vi "Navigate - Base VI For Navigation.vi"(1 "Curr Mining Run":i32=3, 2 "Pathfinding Settings":T1={"Movement Settings"={"Arrival Tolerance (m)"=0.05, "Closeness Threshold (m)"=0.5, "Pit Obstacle Radius (m)"=0.4, "Pit Locations"=[]}, "Dead Zone"=0.9, "Max Moves"=4.0, "Move Segment Length (m)"=0.2, "Path Cost Weights"={"Length Weight"=1.0, "Angle Weight"=0.0, "Angle Error Weight"=150.0, "Angle Error Threshold"=1.04, "Per Move Penalty"=0.25, "Closeness Weight"=3.0, "Too Short Penalty"=100.0, "Too Short Threshold"=1.75}, "Desperation - Reduction Per Attempt (Ratio)"=0.9, "Desperation - Max Attempts"=2, "Log All Move Points"=FALSE, "Intermediate Position Grids"=[{"x1"=0.0, "x2"=4.75, "resolution"=0.45}]}, 3 "Move Type":T5(ring)=enum."Move To Collector Trough") -> ()   [LabVIEW 2015, in "Navigation2017.lvlib"]
uses:
  Navigation2017.lvlib
  PathfindingSettings.ctl
  MovementSettings.ctl
  PathCostWeights.ctl
  IntermediatePositionGrids.ctl
  Vector.ctl
  LocalizationStatus.ctl
  <vilib>/Analysis/coordinate.llb/Angle Units.ctl
  PathOfMoves.ctl
  Move.ctl
  <vilib>/Analysis/coordinate.llb/Absolute Angle Difference (scalar).vi
  <vilib>/Analysis/coordinate.llb/Wrap Angle (scalar).vi
  <vilib>/Analysis/coordinate.llb/Set Angle Unit.vi
  Types - Navigation2017.lvlib
  SubVIs - Navigation2017.lvlib
  Util - Navigation2017.lvlib
  TestbenchUtils - Navigation2017.lvlib
  <vilib>/Analysis/NI_AAL_Angle.lvlib
panel:
  in  "Reached Next Path Point Threshold Angle (rad)":dbl(knob)=1.5491432484410714 scale=0.0..3.14
  out "Pathfinding Loop Count":i32=1
  in  "Reached Next Path Point Threshold Distance (m)":dbl(knob)=0.4892209620058784 scale=0.0..1.0
  in  "Robot Speed":dbl(slide)=1.0 scale=0.0..1.0
  in  "Dead Reckoning Move Distance (m)":dbl(knob)=1.4397205209376083 scale=0.5..4.0
  in  "Turning Radius (m)":dbl(knob)=2.2057844750732873 scale=0.75..4.0
  # "NOTE: Log All Move Points is ignored and\nautomatically switched off."
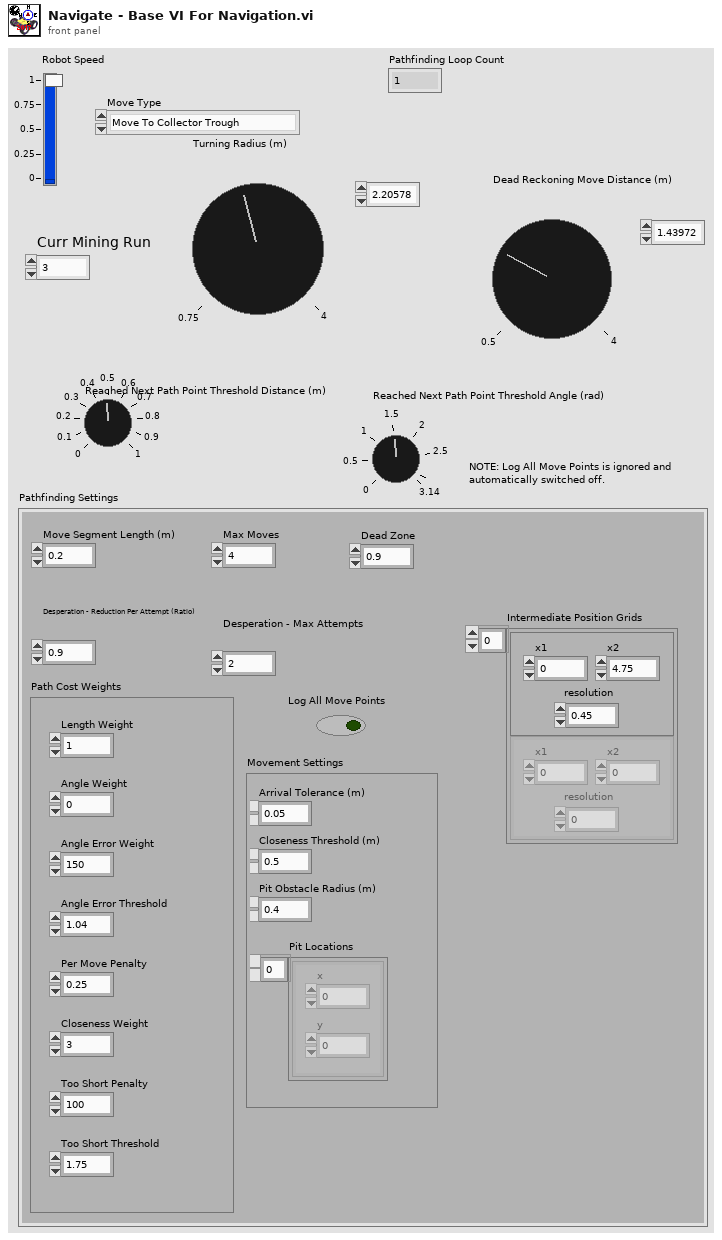
[diagram p1: front panel]
types:
  T1 = typedef "Navigation2017.lvlib/Types - Navigation2017.lvlib/PathfindingSettings.ctl" = cluster{"Movement Settings":T2, "Dead Zone":dbl, "Max Moves":dbl, "Move Segment Length (m)":dbl, "Path Cost Weights":T3, "Desperation - Reduction Per Attempt (Ratio)":dbl, "Desperation - Max Attempts":i16, "Log All Move Points":bool, "Intermediate Position Grids":T4}
  T2 = typedef "Navigation2017.lvlib/Types - Navigation2017.lvlib/MovementSettings.ctl" = cluster{"Arrival Tolerance (m)":dbl, "Closeness Threshold (m)":dbl, "Pit Obstacle Radius (m)":dbl, "Pit Locations":cluster{"x":dbl, "y":dbl}[]}
  T3 = typedef "Navigation2017.lvlib/Types - Navigation2017.lvlib/PathCostWeights.ctl" = cluster{"Length Weight":dbl, "Angle Weight":dbl, "Angle Error Weight":dbl, "Angle Error Threshold":dbl, "Per Move Penalty":dbl, "Closeness Weight":dbl, "Too Short Penalty":dbl, "Too Short Threshold":dbl}
  T4 = typedef "Navigation2017.lvlib/Types - Navigation2017.lvlib/IntermediatePositionGrids.ctl" = cluster{"x1":dbl, "x2":dbl, "resolution":dbl}[]
  T5 = enum16{"Spin and Move To Mining Area", "Move To Collector Trough", "Move To Mining Area"}
  T6 = typedef "Navigation2017.lvlib/Types - Navigation2017.lvlib/Vector.ctl" = cluster{"x":dbl, "y":dbl, "angle":dbl}
  T7 = typedef "Navigation2017.lvlib/TestbenchUtils - Navigation2017.lvlib/LocalizationStatus.ctl" = cluster{"x":dbl, "y":dbl, "angle":dbl, "valid":bool, "lastUpdatedTime":dbl}
  T8 = typedef "Navigation2017.lvlib/Types - Navigation2017.lvlib/PathOfMoves.ctl" = cluster{"Dest Angle Error":dbl, "Dest Angle Considered":bool, "Moves":T9[]}
  T9 = typedef "Navigation2017.lvlib/Types - Navigation2017.lvlib/Move.ctl" = cluster{"Did Reach Dest":bool, "Did Collide":bool, "Sum of Angle Changes (rad)":dbl, "Move Length (m)":dbl, "Closeness Sum":dbl, "Positions Along Move":T6[], "Moved Fwd":bool}
  T10 = typedef "NI_AAL_Angle.lvlib/Angle Units.ctl" = i32
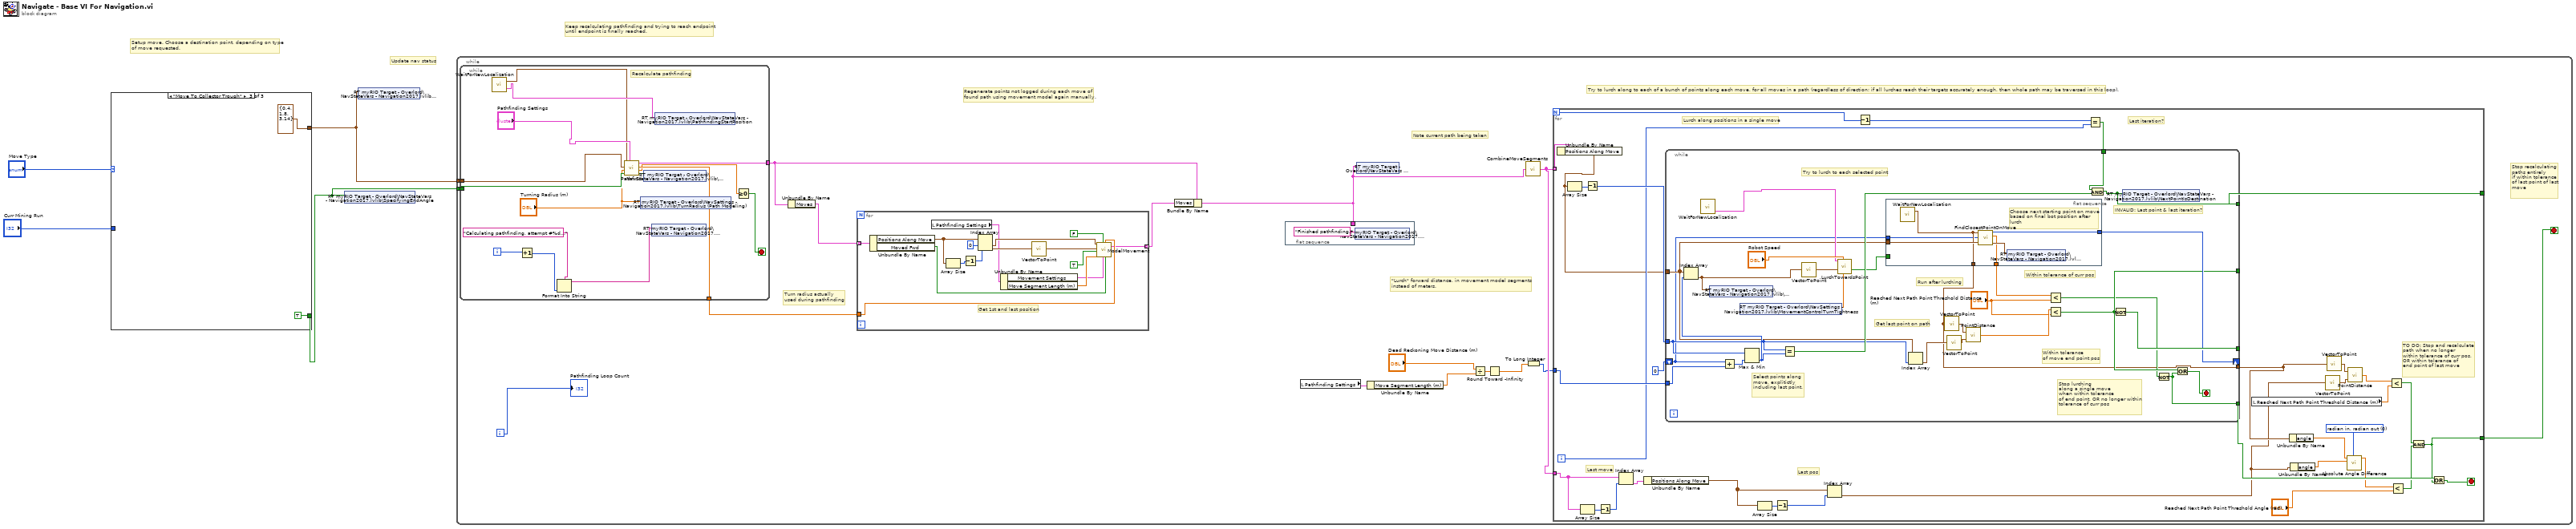
[diagram p0: block diagram]
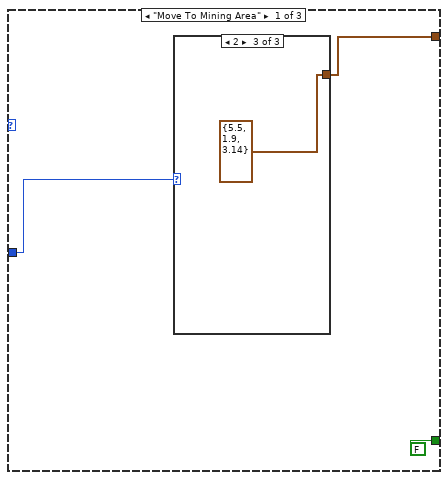
[diagram p2: hidden frame]
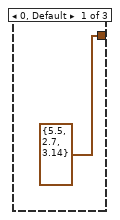
[diagram p3: hidden frame]
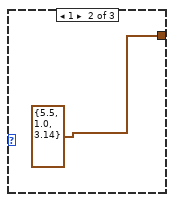
[diagram p4: hidden frame]
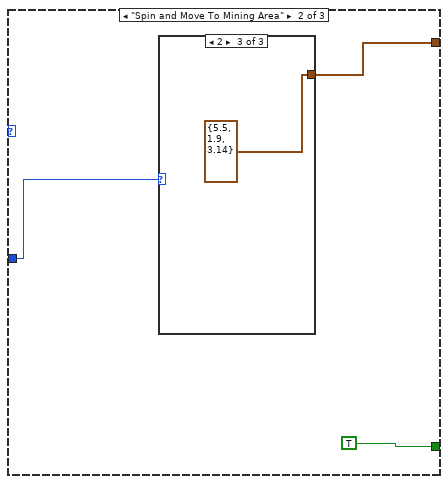
[diagram p5: hidden frame]
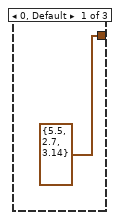
[diagram p6: hidden frame]
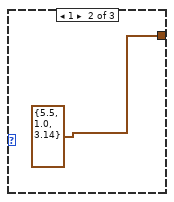
[diagram p7: hidden frame]
diagram:
  # "Keep recalculating pathfinding and trying to reach endpoint\nuntil endpoint is finally reached."
  # "Update nav status"
  # "Setup move. Choose a destination point, depending on type\nof move requested."
  n1 = case shown="\"Move To Collector Trough\"" "Move Type" {
    tunnel: [w5 w12 T6 {"x"=0.4, "y"=1.8, "angle"=3.14} ("Vector")] -> w3
    tunnel: [FALSE TRUE TRUE] -> w2
    tunnel: "Curr Mining Run" -> [w6 w11 _]
    frame "Move To Mining Area" {
      n2 = case shown="2" w6 {
        tunnel: [T6 {"x"=5.5, "y"=2.7, "angle"=3.14} ("Vector") T6 {"x"=5.5, "y"=1.0, "angle"=3.14} ("Vector") T6 {"x"=5.5, "y"=1.9, "angle"=3.14} ("Vector")] -> w5
        frame 0, Default {
        }
        frame 1 {
        }
        frame 2 {
        }
      }
    }
    frame "Spin and Move To Mining Area" {
      n3 = case shown="2" w11 {
        tunnel: [T6 {"x"=5.5, "y"=2.7, "angle"=3.14} ("Vector") T6 {"x"=5.5, "y"=1.0, "angle"=3.14} ("Vector") T6 {"x"=5.5, "y"=1.9, "angle"=3.14} ("Vector")] -> w12
        frame 0, Default {
        }
        frame 1 {
        }
        frame 2 {
        }
      }
    }
    frame "Move To Collector Trough" {
    }
  }
  n4 = shared-variable "RT myRIO Target - Overlord\\NavStateVars - Navigation2017.lvlib\\SpecifyingEndAngle"(w2) -> ()  [unwired: 1 in, 1 out]
  n5 = shared-variable "RT myRIO Target - Overlord\\NavStateVars - Navigation2017.lvlib\\DestinationPoint"(w3) -> ()  [unwired: 1 in, 1 out]
  n6 = while {
    tunnel: w3 -> [w33]
    tunnel: w2 -> [w32]
    i -> [w34]
    stop <- w21 stop-if-true
    # "Stop recalculating\npaths entirely\nif within tolerance\nof last point of last\nmove"
    # "Try to lurch along to each of a bunch of points along each move, for all moves in a path (regardless of direction; if all lurches reach their targets accurately enough, then whole path may be traversed in this loop)."
    # "Turn radius actually\nused during pathfinding"
    # "Regenerate points not logged during each move of\nfound path using movement model again manually."
    # "\"Lurch\" forward distance, in movement model segments\ninstead of meters."
    # "Note current path being taken"
    n7 = while {
      tunnel: w33 -> [w49]
      tunnel: w32 -> [w48]
      tunnel: [w45] -> w27
      tunnel: [w43] -> w24
      i -> [w38]
      stop <- w39 stop-if-true
      # "Recalculate pathfinding"
      n8 = call "WaitForNewLocalization.vi"() -> ("Localization Status"=w46:T7, "Localization Status Vector"=w41:T6)
      n9 = Increment(x=w38) -> (x+1=w36:i32)
      n10 = Format Into String(format string="Calculating pathfinding, attempt #%d..." ("CurrNavStage"), w36) -> (resulting string=w35:string)  [unwired: 2 in, 1 out]
      n11 = call "Pathfind.vi"("Pathfinding Settings"="Pathfinding Settings", "Specified End Angle"=w48, "Turn Radius (m)"="Turning Radius (m)", "Destination"=w49, "Start Vector"=w41) -> ("Desperation Used"=w47:bool, "Total Paths Arrived"=w40:dbl, "Used Turn Radius (m)"=w45:dbl, "Best Path"=w43:T8)  [unwired: 1 out]
      n12 = shared-variable "RT myRIO Target - Overlord\\NavSettings - Navigation2017.lvlib\\TurnRadius (Path Modeling)"("Turning Radius (m)") -> ()  [unwired: 1 in, 1 out]
      n13 = shared-variable "RT myRIO Target - Overlord\\NavStateVars - Navigation2017.lvlib\\UsedDesperation"(w47) -> ()  [unwired: 1 in, 1 out]
      n14 = shared-variable "RT myRIO Target - Overlord\\NavStateVars - Navigation2017.lvlib\\CurrNavStage"(w35) -> ()  [unwired: 1 in, 1 out]
      n15 = shared-variable "RT myRIO Target - Overlord\\NavStateVars - Navigation2017.lvlib\\PathfindingStartPosition"(w46) -> ()  [unwired: 1 in, 1 out]
      n16 = Greater Or Equal To 0?(x=w40) -> (x >= 0?=w39:bool)
    }
    n17 = Unbundle By Name(w24) -> ("Moves"=w26:T9[])
    n18 = for {
      tunnel: w27 -> [w66]
      tunnel: w26 -> [w65] mode=indexing
      tunnel: [w55] -> w25 mode=indexing
      # "Get 1st and last position"
      n19 = Unbundle By Name(w65) -> ("Positions Along Move"=w53:T6[], "Moved Fwd"=w64:bool)
      n20 = local read "Pathfinding Settings"() -> (w58:T1)
      n21 = Array Size(array=w53) -> (size(s)=w52:i32)
      n22 = Decrement(x=w52) -> (x-1=w51:i32)
      n23 = Index Array(array=w53, index #1=0 ("index"), index #2=w51) -> (element #1=w62:T6, element #2=w60:T6)
      n24 = Unbundle By Name(w58) -> ("Movement Settings"=w56:T2, "Move Segment Length (m)"=w57:dbl)
      n25 = call "VectorToPoint.vi"("Vector"=w60) -> ("Point"=w61:cluster{"x":dbl, "y":dbl})
      n26 = call "ModelMovement.vi"("Start Vector"=w62, "Destination"=w61, "Log All Points"=TRUE, "Segment Length (m)"=w57, "Do Force Direction"=FALSE, "Movement Settings"=w56, "Turn Radius (m)"=w66, "Force Direction Forward (If Forcing)"=w64) -> ("Move"=w55:T9)  [unwired: 10 in, 1 out]
    }
    n27 = Bundle By Name(cluster=w24, "Moves"=w25) -> (w23:T8)
    n28 = flat-sequence {
      tunnel: w23 -> [_]
      frame #0 {
        n29 = shared-variable "RT myRIO Target - Overlord\\NavStateVars - Navigation2017.lvlib\\CurrNavStage"("Finished pathfinding." ("CurrNavStage")) -> ()  [unwired: 1 in, 1 out]
      }
    }
    n30 = local read "Pathfinding Settings"() -> (w28:T1)
    n31 = shared-variable "RT myRIO Target - Overlord\\NavStateVars - Navigation2017.lvlib\\CurrPath"(w23) -> ()  [unwired: 1 in, 1 out]
    n32 = Unbundle By Name(w28) -> ("Move Segment Length (m)"=w29:dbl)
    n33 = Divide(x="Dead Reckoning Move Distance (m)", y=w29) -> (x/y=w31:dbl)
    n34 = Round Toward -Infinity(1:w31) -> (0:w20:dbl)
    n35 = call "CombineMoveSegments.vi"("Path"=w23) -> ("Combined Moves (Discarding Metadata Save Moved Fwd)"=w22:T9[])
    n36 = To Long Integer(number=w20) -> (32bit integer=w19:i32)
    n37 = for {
      N -> [w96]
      tunnel: w19 -> [w100]
      tunnel: [w92] -> _
      tunnel: w22 -> [w83] mode=indexing
      tunnel: w22 -> [w86]
      tunnel: [w75] -> w21
      i -> [w94]
      stop <- w89 stop-if-true
      w72 = T10 0 items=["radian in, radian out", "radian in, degree out", "degree in, degree out", "degree in, radian out"] ("angle units")
      # "Last pos"
      # "Last move"
      # "Lurch along positions in a single move"
      # "TO DO: Stop and recalculate\npath when no longer\nwithin tolerance of curr pos, \nOR within tolerance of \nend point of last move"
      # "Last iteration?"
      n38 = Unbundle By Name(w83) -> ("Positions Along Move"=w82:T6[])
      n39 = Array Size(array=w82) -> (size(s)=w98:i32)
      n40 = Array Size(array=w86) -> (size(s)=w80:i32)
      n41 = Decrement(x=w98) -> (x-1=w97:i32)
      n42 = Decrement(x=w80) -> (x-1=w79:i32)
      n43 = Index Array(array=w86, index=w79) -> (element=w78:T9)
      n44 = Unbundle By Name(w78) -> ("Positions Along Move"=w81:T6[])
      n45 = Array Size(array=w81) -> (size(s)=w85:i32)
      n46 = Decrement(x=w85) -> (x-1=w77:i32)
      n47 = Index Array(array=w81, index=w77) -> (element=w69:T6)
      n48 = Decrement(x=w96) -> (x-1=w95:i32)
      n49 = Equal?(x=w95, y=w94) -> (x = y?=w93:bool)
      n50 = while {
        shift-right: [w115] -> _
        shift-left: i16 0 -> [w101]
        tunnel: w100 -> [w128]
        tunnel: w97 -> [w113]
        tunnel: w82 -> [w112]
        tunnel: [w123] -> _
        tunnel: w93 -> [w121]
        tunnel: [w120] -> w92
        tunnel: [w105] -> _
        tunnel: [w103] -> w91
        tunnel: [w102] -> w70
        stop <- w124 stop-if-true
        # "Within tolerance of curr pos"
        # "Get last point on path"
        # "Stop lurching\nalong a single move\nwhen within tolerance\nof end point, OR no longer within\ntolerance of curr pos"
        # "Within tolerance\nof move end point pos"
        # "Run after lurching"
        # "Select points along\nmove, explitictly including last point."
        # "INVALID: Last point & last iteration?"
        # "Try to lurch to each selected point"
        n51 = call "WaitForNewLocalization.vi"() -> ("Localization Status"=w117:T7)  [unwired: 1 out]
        n52 = Add(x=w101, y=w128) -> (x+y=w127:i32)
        n53 = shared-variable "RT myRIO Target - Overlord\\NavSettings - Navigation2017.lvlib\\MovementControlTurnTightness"() -> (w118:dbl)  [unwired: 1 in, 1 out]
        n54 = Max & Min(x=w113, y=w127) -> (min(x,y)=w116:i32)  [unwired: 1 out]
        n55 = Index Array(array=w112, index=w116) -> (element=w119:T6)
        n56 = shared-variable "RT myRIO Target - Overlord\\NavStateVars - Navigation2017.lvlib\\NextPointOnPath"(w119) -> ()  [unwired: 1 in, 1 out]
        n57 = Equal?(x=w113, y=w116) -> (x = y?=w122:bool)
        n58 = call "VectorToPoint.vi"("Vector"=w119) -> ("Point"=w126:cluster{"x":dbl, "y":dbl})
        n59 = call "LurchTowardsPoint.vi"("Turning Radius (m) \n(Goes into Dillons' Movement Control)"=w118, "Robot Speed"="Robot Speed", "Dest. Point"=w126, "Curr Localization Status"=w117) -> ("Within Tolerance of Dest (DEPRECATED AND BROKEN)"=w114:bool)  [unwired: 2 in, 1 out]
        n60 = flat-sequence {
          tunnel: w112 -> [w134]
          tunnel: [w132] -> w115
          tunnel: w114 -> [_]
          tunnel: [w130] -> w102
          tunnel: [w131] -> w106
          tunnel: w101 -> [w129]
          frame #0 {
            # "Choose next starting point on move\nbased on final bot position after\nlurch"
            n61 = call "WaitForNewLocalization.vi"() -> ("Localization Status Vector"=w130:T6)  [unwired: 1 out]
            n62 = call "FindClosestPointOnMove.vi"("Current Robot Position"=w130, "Start Index"=w129, "Move Positions"=w134) -> ("Closest Index"=w132:i32, "Coordinate Error"=w131:dbl, "Closest Vector"=w133:T6)  [unwired: 1 out]
            n63 = shared-variable "RT myRIO Target - Overlord\\NavStateVars - Navigation2017.lvlib\\CurrPosOnPath"(w133) -> ()  [unwired: 1 in, 1 out]
          }
        }
        n64 = Index Array(array=w112, index=w113) -> (element=w111:T6)
        n65 = call "VectorToPoint.vi"("Vector"=w102) -> ("Point"=w109:cluster{"x":dbl, "y":dbl})
        n66 = call "VectorToPoint.vi"("Vector"=w111) -> ("Point"=w110:cluster{"x":dbl, "y":dbl})
        n67 = call "PointDistance.vi"("Point 2"=w110, "Point 1"=w109) -> ("Distance"=w108:dbl)
        n68 = Less?(x=w106, y="Reached Next Path Point Threshold Distance (m)") -> (x < y?=w104:bool)
        n69 = Less?(x=w108, y="Reached Next Path Point Threshold Distance (m)") -> (x < y?=w105:bool)
        n70 = And(x=w121, y=w122) -> (x .and. y?=w120:bool)
        n71 = Not(x=w105) -> (.not. x?=w123:bool)
        n72 = shared-variable "RT myRIO Target - Overlord\\NavStateVars - Navigation2017.lvlib\\NextPointIsDestination"(w120) -> ()  [unwired: 1 in, 1 out]
        n73 = Not(x=w104) -> (.not. x?=w103:bool)
        n74 = Or(x=w105, y=w103) -> (x .or. y?=w124:bool)
      }
      n75 = local read "Reached Next Path Point Threshold Distance (m)"() -> (w90:dbl)
      n76 = Unbundle By Name(w70) -> ("angle"=w67:dbl)
      n77 = Unbundle By Name(w69) -> ("angle"=w68:dbl)
      n78 = call "VectorToPoint.vi"("Vector"=w69) -> ("Point"=w84:cluster{"x":dbl, "y":dbl})
      n79 = call "VectorToPoint.vi"("Vector"=w70) -> ("Point"=w88:cluster{"x":dbl, "y":dbl})
      n80 = call-poly <vilib>:"Absolute Angle Difference.vi"("angle units"=w72, "angle 2"=w68, "angle 1"=w67) -> ("absolute angle difference"=w71:dbl)  [unwired: 7 in, 1 out]
      n81 = call "PointDistance.vi"("Point 2"=w84, "Point 1"=w88) -> ("Distance"=w87:dbl)
      n82 = Less?(x=w87, y=w90) -> (x < y?=w74:bool)
      n83 = Less?(x=w71, y="Reached Next Path Point Threshold Angle (rad)") -> (x < y?=w73:bool)
      n84 = And(x=w74, y=w73) -> (x .and. y?=w75:bool)
      n85 = Or(x=w91, y=w75) -> (x .or. y?=w89:bool)
    }
    "Pathfinding Loop Count" <- w34
  }
